vi "AdminLogon.vi"(8 "ErrorIn":errorcluster, 11 "Password":string) -> (0 "ErrorOut":errorcluster, 3 "Successful?":bool)   [LabVIEW 2018]
doc: "This modal dialog allows administrative-level users to enter a password to unlock privileged features of the application. This is used in conjunction with the UserLevelEnum TypeDef control.\n\nCopyright © 2019 Epimedia, Inc. All Rights Reserved.\n\nThe Epimedia Application Library is Copyright © 2009-2019 Epimedia, Inc. \nAll Rights Reserved. Used under license."
panel:
  out "Error":string="Incorrect Password!!"
  in  "Cancel":bool
  in  "OK":bool
  in  "Password":string
  # "Enter Adminstrator Password :"
  # "Copyright © 2019 Epimedia, Inc. All Rights Reserved.\n\nThe Epimedia Application Library is Copyright © 2009-2019 Epimedia, Inc. \nAll Rights Reserved. Used under license."
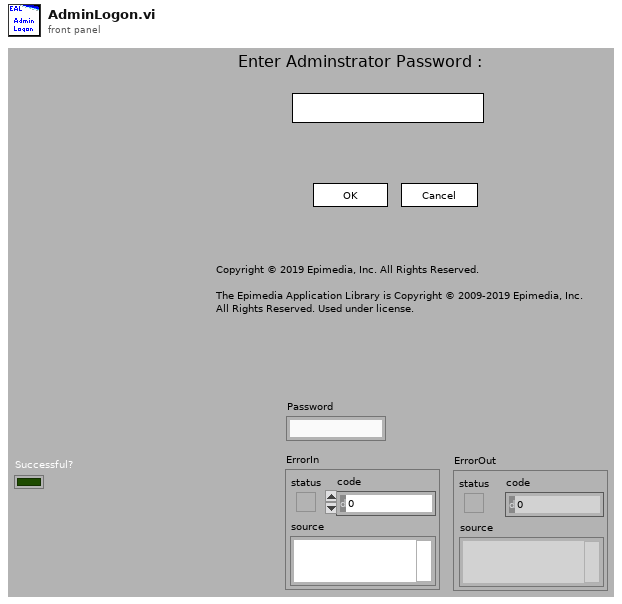
[diagram p1: front panel]
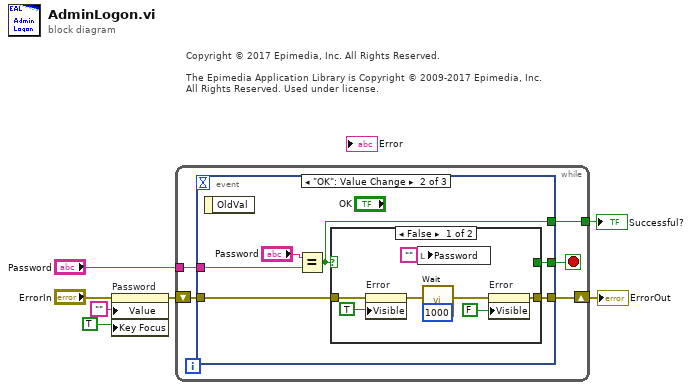
[diagram p0: block diagram]
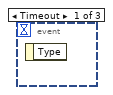
[diagram p2: hidden frame]
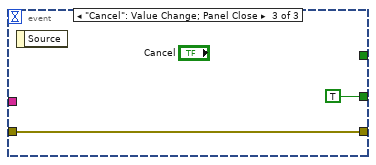
[diagram p4: hidden frame]
diagram:
  # "Copyright © 2017 Epimedia, Inc. All Rights Reserved.\n\nThe Epimedia Application Library is Copyright © 2009-2017 Epimedia, Inc. \nAll Rights Reserved. Used under license."
  n1 = property on="Password" class="Str"(error in="ErrorIn", "Value"="" ("Password"), "Key Focus"=TRUE) -> (error out=w6:errorcluster)  [unwired: 1 in, 1 out]
  n2 = while {
    shift-right: [w9] -> w3
    shift-left: w6 -> [w12]
    tunnel: [w11] -> w7
    tunnel: "Password" -> [w8]
    stop <- w10 stop-if-true
    n3 = event shown="[1] \"OK\": Value Change" {
      selector: _ -> [_ _ _]
      dyn-events: _ -> [_ _ _]
      timeout: _ -> [_ _ _]
      tunnel: w12 -> [_ w18 w29]
      tunnel: [_ w17 w29] -> w9
      tunnel: [_ w16 _] -> w11
      tunnel: [_ w15 TRUE] -> w10
      tunnel: w8 -> [_ w13 _]
      event Timeout {
        n4 = event-data() -> ()  [unwired: 2 out]
      }
      event "OK": Value Change {
        n5 = event-data() -> ()  [unwired: 2 out]
        n6 = Equal?(x="Password", y=w13) -> (x = y?=w16:bool)
        n7 = case shown="False" w16 {
          selector: w16 -> [_ w27]
          tunnel: w18 -> [w26 w28]
          tunnel: [w23 w28] -> w17
          tunnel: [_ w27] -> w15
          frame False {
            n8 = property on="Error" class="Str"(error in=w26, "Visible"=TRUE) -> (error out=w22:errorcluster)  [unwired: 1 in, 1 out]
            n9 = local write "Password"("" ("Password")) -> ()
            n10 = call "Wait.vi"("Wait (ms)"=u32 1000, "ErrorIn"=w22) -> ("ErrorOut"=w21:errorcluster)  [unwired: 9 in]
            n11 = property on="Error" class="Str"(error in=w21, "Visible"=FALSE) -> (error out=w23:errorcluster)  [unwired: 1 in, 1 out]
          }
          frame True {
          }
        }
      }
      event "Cancel": Value Change; Panel Close {
        n12 = event-data() -> ()  [unwired: 2 out]
      }
    }
  }
  "ErrorOut" <- w3
  "Successful?" <- w7
